vi "_DServerLog.vi"(3 "text":string="unspecified_log_text", 4 "device name":string="unspecified_device_name", 5 "logging level":T1) -> ()   [LabVIEW 2014, in "tango.lvlib"]
uses:
  tango.lvlib
  _LoggingLevel.ctl
  tango_binding.so
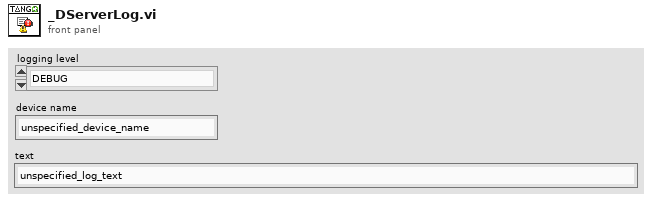
[diagram p1: front panel]
types:
  T1 = typedef "tango.lvlib/_LoggingLevel.ctl" = enum16{"DEBUG", "INFO", "WARNING", "ERROR", "FATAL"}
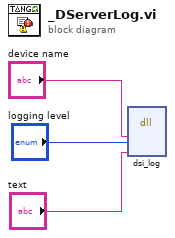
[diagram p0: block diagram]
diagram:
  n1 = dll-call lib="tango_binding.*" fn="dsi_log"("device_name"="device name", "level"="logging level", "text"="text") -> ()  [unwired: 7 in, 2 out]
